vi "sub_img_process_main.vi"(8 "error in":errorcluster, 10 "Image Dst":T1=refnum, 11 "Image Src":T1=refnum) -> (0 "error out":errorcluster, 1 "Edge Coordinates":cluster{"X":sgl, "Y":sgl}[](array[cluster])=[{"X"=395.02045, "Y"=323.0}, {"X"=608.6168, "Y"=323.0}] {"Y" format="%.2f"; "X" format="%.2f"}, 2 "dir-data":cluster{"Distance":sgl, "weight-dir":dbl}={"Distance"=213.59637, "weight-dir"=-10.181365966796875}, 3 "Image roi-in":T1(plugin-control))   [LabVIEW 2019]
uses:
  <vilib>/vision/Image Controls.llb/IMAQ Image.ctl
  Ctrl/clamp-result_cmd.ctl
  <vilib>/vision/NI_Vision_Development_Module.lvlib
panel:
  out "Distance":sgl=780.4965 format="%.2f"
  in  "Tab Control":enum32{"Clamp", "io"}(tab)
  out "웨이브폼 차트":sgl(graph)=780.4965
  out "Image":T1(plugin-control)
  in  "Color Plane":i32(ring)=1 items=["Red", "Green", "Blue", "Hue", "Saturation", "Luminance", "Value", "Intensity"]
  in  "Clamp Settings":T2={"Contrast"=20, "Filter width"=4, "Steepness"=2, "Subsampling Ratio"=5, "Show Search Area"=TRUE, "Show Search Lines"=TRUE, "Show Edges Found"=TRUE, "Show Result"=TRUE}
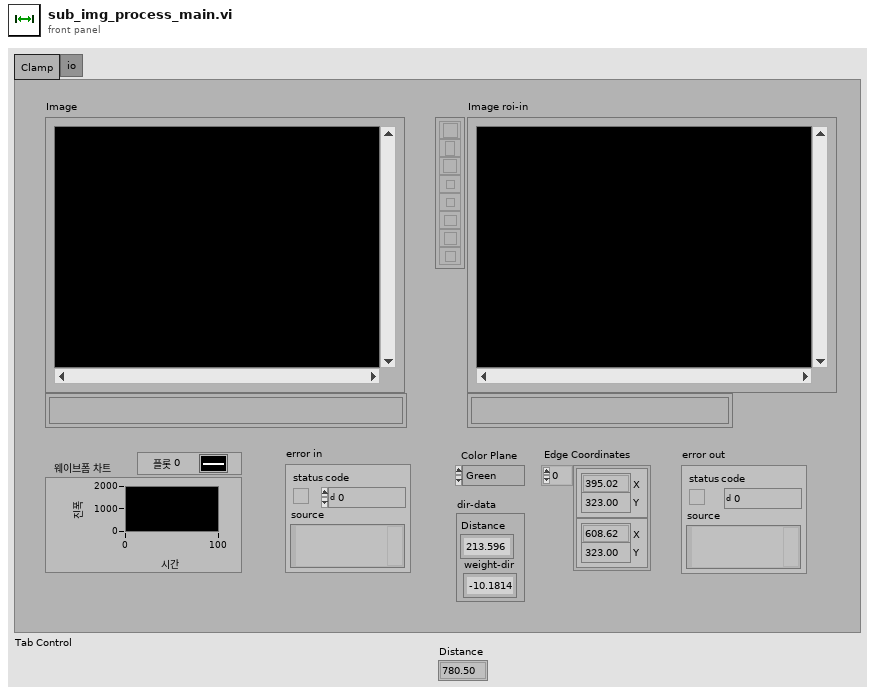
[diagram p1: front panel]
types:
  T1 = typedef "IMAQ Image.ctl" = refnum<image>
  T2 = cluster{"Contrast":i32, "Filter width":i32, "Steepness":i32, "Subsampling Ratio":u32, "Show Search Area":bool, "Show Search Lines":bool, "Show Edges Found":bool, "Show Result":bool}
  T3 = typedef "clamp-result_cmd.ctl" = enum16{"write_clamp_overlay-result", "write_center-distance", "write_clamp_result", "write_threshold_result", "read"}
  T4 = cluster{"Global Rectangle":i32[], "Contours":cluster{"Contour Type":u32, "ROI Type":u32, "Points":i32[]}[]}
  T5 = typedef "IMAQ Rectangle" = cluster{"Left":i32, "Top":i32, "Right":i32, "Bottom":i32, "Rotation":dbl}
  T6 = cluster{"Clamp Settings":cluster{"Contrast":i32, "Filter width":i32, "Steepness":i32, "Subsampling Ratio":u32, "Show Search Area":bool, "Show Search Lines":bool, "Show Edges Found":bool, "Show Result":bool}, "Range":cluster{"Lower value":sgl, "Upper value":sgl}, "N of Erosion 1":i32, "N of Erosion 2":i32}
  T7 = typedef "ROI Descriptor" = cluster{"Global Rectangle":i32[], "Contours":cluster{"ID":enum32{"External", "Internal"}, "Type":u32, "Coordinates":i32[]}[]}
  T8 = cluster{"Points":cluster{"X":sgl, "Y":sgl}[], cluster{"X":sgl, "Y":sgl}[], cluster{cluster{"X":sgl, "Y":sgl}, cluster{"X":sgl, "Y":sgl}}[], "Perpendicular Lines":cluster{cluster{"X":sgl, "Y":sgl}, cluster{"X":sgl, "Y":sgl}}[], "ROI Descriptor out":T7}
  T9 = cluster{"Edge Coordinates":cluster{"X":sgl, "Y":sgl}[], "dir-data":cluster{"Distance":sgl, "weight-dir":dbl}, "clamp_result":cluster{"Points":cluster{"X":sgl, "Y":sgl}[], cluster{"X":sgl, "Y":sgl}[], cluster{cluster{"X":sgl, "Y":sgl}, cluster{"X":sgl, "Y":sgl}}[], "Perpendicular Lines":cluster{cluster{"X":sgl, "Y":sgl}, cluster{"X":sgl, "Y":sgl}}[], "ROI Descriptor out":T7}}
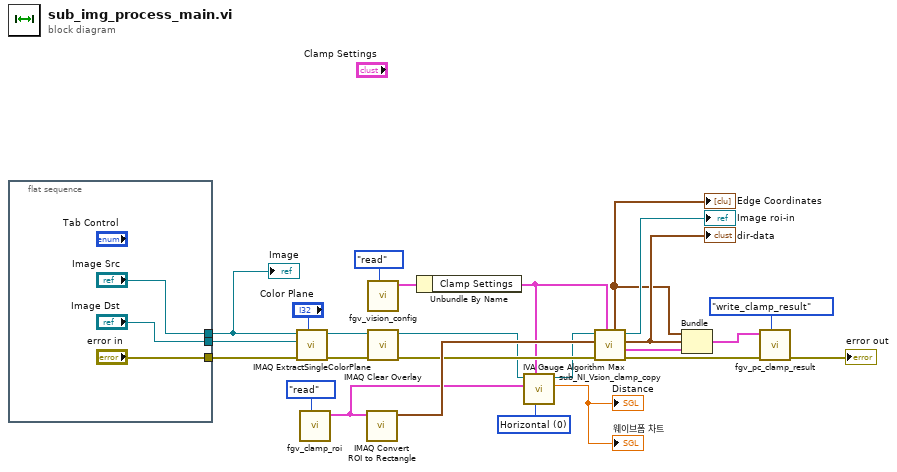
[diagram p0: block diagram]
diagram:
  w8 = u32 0 items=["Horizontal", "Vertical"] ("Scanning axis (Clamp (Rake) 1)")
  n1 = flat-sequence {
    tunnel: ["error in"] -> w15
    tunnel: ["Image Dst"] -> w16
    tunnel: ["Image Src"] -> w11
    frame #0 {
    }
  }
  n2 = call "IMAQ ExtractSingleColorPlane"("Color Plane"="Color Plane", "error in (no error)"=w15, "Image Dst"=w16, "Image Src"=w11) -> ("error out"=w20:errorcluster, "Image Dst Out"=w19:T1)  [unwired: 6 in]
  n3 = call "fgv_clamp_roi.vi"("cmd"=enum16{"init", "read", "write"}."read") -> ("ROI-clamp out"=w6:T4)  [unwired: 10 in]
  n4 = call "IMAQ Convert ROI to Rectangle"("ROI Descriptor"=w6) -> ("Rectangle"=w24:T5)  [unwired: 8 in, 1 out]
  n5 = call "fgv_vision_config.vi"("cmd"=enum16{"init", "read", "write"}."read") -> ("Vison cfg out"=w7:T6)  [unwired: 9 in, 1 out]
  n6 = call "IMAQ Clear Overlay"("error in (no error)"=w20, "Image"=w19) -> ("error out"=w21:errorcluster, "Image Out"=w5:T1)  [unwired: 8 in]
  n7 = Unbundle By Name(w7) -> ("Clamp Settings"=w2:T2)
  n8 = call <vilib>:"IVA Gauge Algorithm Max.vi"("Scanning axis"=w8, "Settings"=w2, "ROI Descriptor"=w6, "Image"=w5) -> ("Distance"=→"Distance" →"웨이브폼 차트":sgl, "Image Out"=w4:T1)  [unwired: 2 in, 4 out]
  n9 = call "sub_NI_Vsion_clamp_copy.vi"("Settings"=w2, "error in (no error)"=w21, "Rectangle"=w24, "Image"=w4) -> ("error out"=w18:errorcluster, "clamp_result"=w22:T8, "dir-data"=w13:cluster{"Distance":sgl, "weight-dir":dbl}, "Image Out"=→"Image roi-in":T1, "Edge Coordinates"=w1:cluster{"X":sgl, "Y":sgl}[])  [unwired: 3 in]
  "Edge Coordinates" <- w1
  "dir-data" <- w13
  n10 = Bundle("Edge Coordinates"=w1, "dir-data"=w13, "clamp_result"=w22) -> (w12:T9)  [unwired: 1 in]
  n11 = call "fgv_pc_clamp_result.vi"("cmd"=clamp-result_cmd."write_clamp_result", "error in"=w18, "clamp result in"=w12) -> ("error out"=→"error out":errorcluster)  [unwired: 5 in, 3 out]
  "Image" <- w11
